vi "Read Color.vi"(11 "Product In":refnum<class "Product.lvclass">) -> (2 "Color":T1, 3 "Product Out":refnum<class "Product.lvclass">)   [LabVIEW 2018, in "Product.lvclass"]
uses:
  Product.lvclass
  Color.ctl
  Product.lvclass/Product.ctl
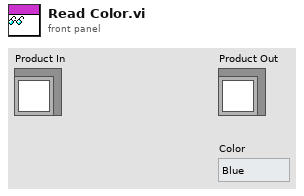
[diagram p1: front panel]
types:
  T1 = typedef "Product.lvclass/Color.ctl" = enum16{"Blue", "Green", "Red"}
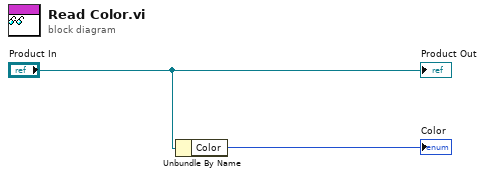
[diagram p0: block diagram]
diagram:
  n1 = Unbundle By Name("Product In") -> ("Color"=→"Color":T1)
  "Product Out" <- "Product In"
